vi "Operator array with space bar continue.vi"(4 "Lower limit":u32=1, 6 "Upper limit":u32=4294967295, 7 "Data format":string="0103ddd", 8 "error in (no error)":errorcluster, 9 "Get decimal response?":bool, 10 "Array":string[][](array[string]), 11 "Message":string) -> (0 "error out":errorcluster, 3 "Decimal response":u32)   [LabVIEW 2013]
uses:
  <vilib>/event_ctls.llb/eventvkey.ctl
panel:
  # "Operator Message"
  # "Press SPACE BAR to continue"
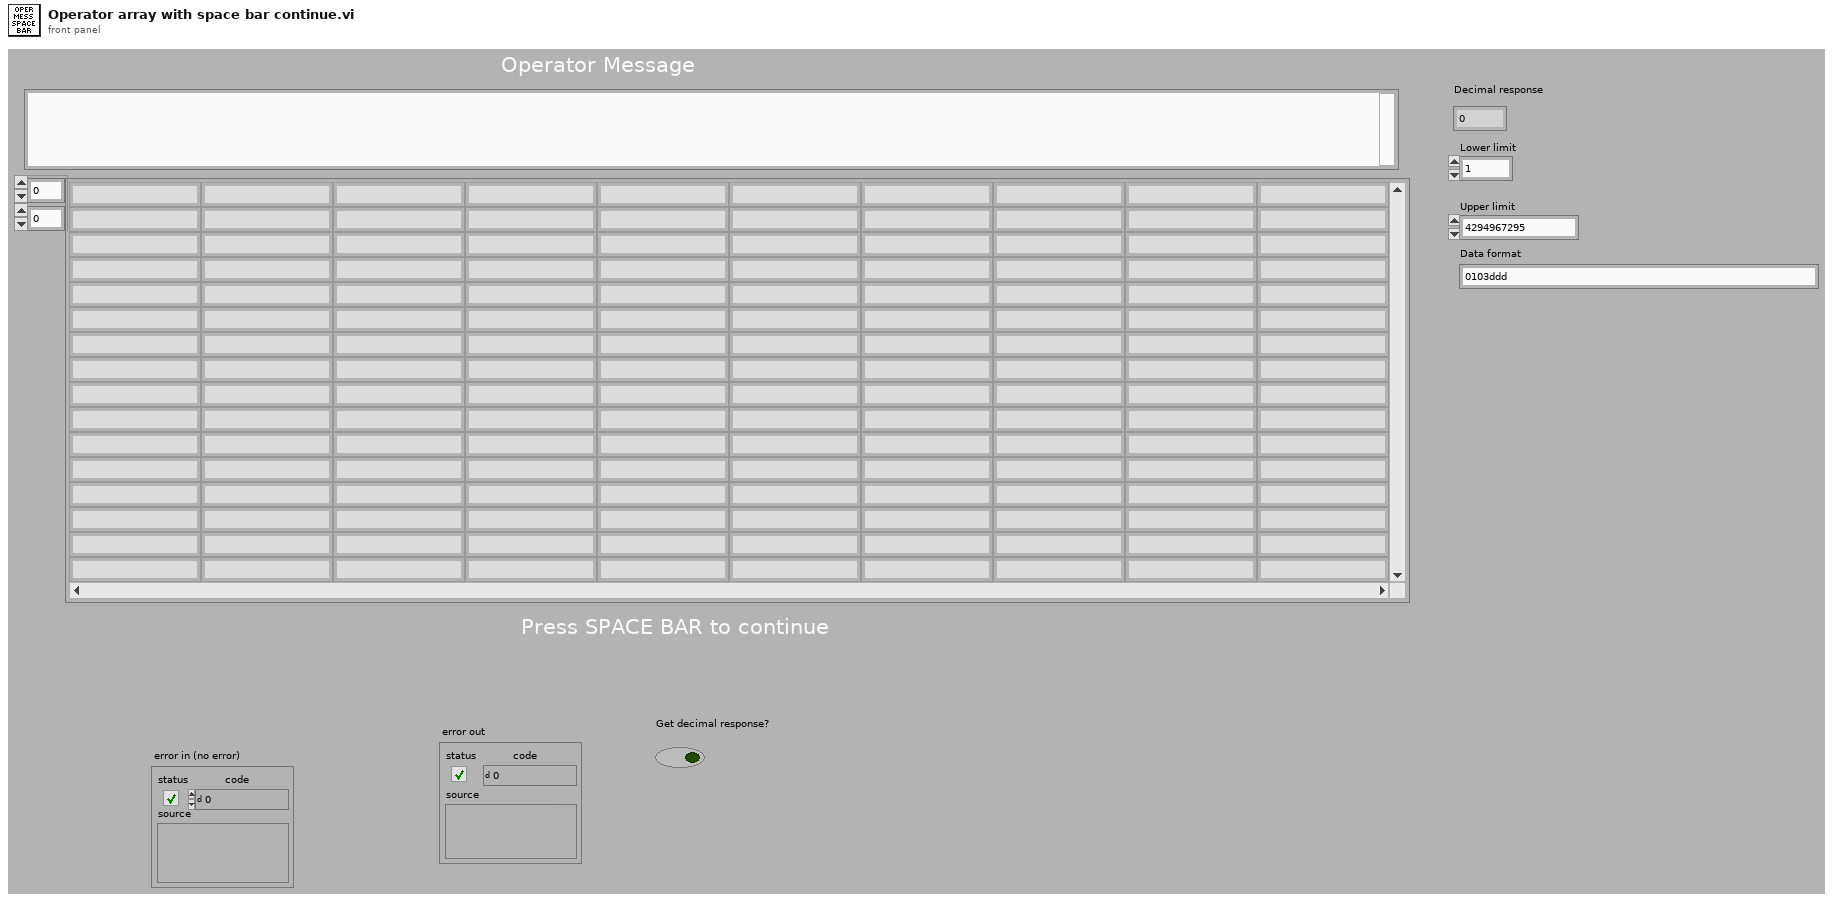
[diagram p1: front panel]
types:
  T1 = typedef "eventvkey.ctl" = enum16{"ASCII", "Enter", "Return", "Shift", "Ctrl", "Alt", "Cmd", "Opt", "Caps", "NumLock", "Clear", "Break", "Up", "Down", "Left", "Right", "Insert", "Delete", "Home", "End", "PageUp", "PageDown", "Escape", "Help", "Pause", "ScrollLock", "F1", "F2", "F3", "F4", "F5", "F6", "F7", "F8", "F9", "F10", "F11", "F12", "F13", "F14", "F15", "F16", "F17", "F18", "F19", "F20", "F21", "F22", "F23", "F24", "Play", "VolumeUp", "VolumeDown", "Mute", "Two Byte Char"}
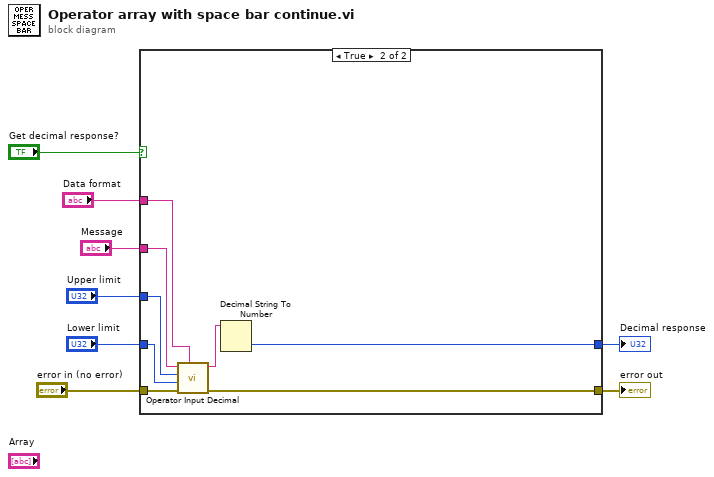
[diagram p0: block diagram]
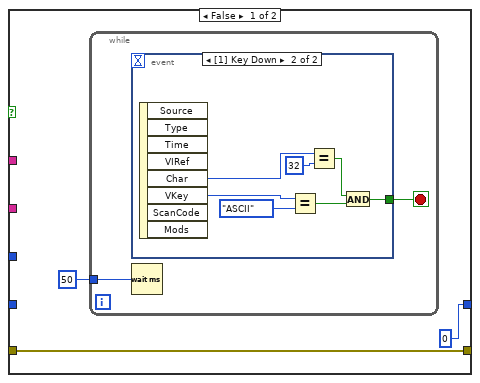
[diagram p2: hidden frame]
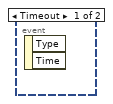
[diagram p3: hidden frame]
diagram:
  n1 = case shown="True" "Get decimal response?" {
    tunnel: "Message" -> [_ w28]
    tunnel: "error in (no error)" -> [w9 w27]
    tunnel: [w9 w26] -> w5
    tunnel: [0 w24] -> w4
    tunnel: "Data format" -> [_ w23]
    tunnel: "Upper limit" -> [_ w22]
    tunnel: "Lower limit" -> [_ w21]
    frame False {
      n2 = while {
        tunnel: u32 50 ("milliseconds to wait") -> [w13]
        stop <- w12 stop-if-true
        n3 = event shown="[1] Key Down" {
          selector: _ -> [_ _]
          dyn-events: _ -> [_ _]
          timeout: _ -> [_ _]
          tunnel: [_ w14] -> w12
          event Timeout {
            n4 = event-data() -> ()  [unwired: 1 in, 2 out]
          }
          event Key Down {
            n5 = event-data() -> ("Char"=w20:i16, "VKey"=w18:T1)  [unwired: 1 in, 6 out]
            n6 = Equal?(x=w18, y=eventvkey."ASCII" ("VKey")) -> (x = y?=w15:bool)
            n7 = Equal?(x=w20, y=i16 32) -> (x = y?=w16:bool)
            n8 = And(x=w16, y=w15) -> (x .and. y?=w14:bool)
          }
        }
        n9 = Wait (ms)(milliseconds to wait=w13) -> ()  [unwired: 1 out]
      }
    }
    frame True {
      n10 = call "Operator Input Decimal.vi"("Data format"=w23, "error in (no error)"=w27, "Lower limit"=w21, "Upper limit"=w22, "Message"=w28) -> ("error out"=w26:errorcluster, "Response"=w25:string)  [unwired: 3 in, 2 out]
      n11 = Decimal String To Number(string=w25) -> (number=w24:i32)  [unwired: 2 in, 1 out]
    }
  }
  "error out" <- w5
  "Decimal response" <- w4
